vi "_012.vi"() -> ()   [LabVIEW 2024]
panel:
  out "output array":dbl[](array[numeric])
  in  "dimension size 2":i32
  in  "array 3":dbl[](array[numeric])
  out "min value":dbl
  out "max index(es)":i32
  out "min index(es)":i32
  out "max value":dbl
  in  "array 2":dbl[](array[numeric])
  out "subarray":dbl[](array[numeric])
  in  "length":i32
  in  "index":i32
  in  "array":dbl[](array[numeric])
  in  "element":dbl
  in  "element":dbl
  in  "element":dbl
  out "appended array":dbl[](array[numeric])
  in  "element":dbl
  out "initialized array":dbl[](array[numeric])
  in  "dimension size":i32
  in  "element":dbl
  # "Array :"
  # "Initilaize Array :"
  # "Build Array :"
  # "Array Subset :"
  # "Reshape Array :"
  # "Array Max & Min :"
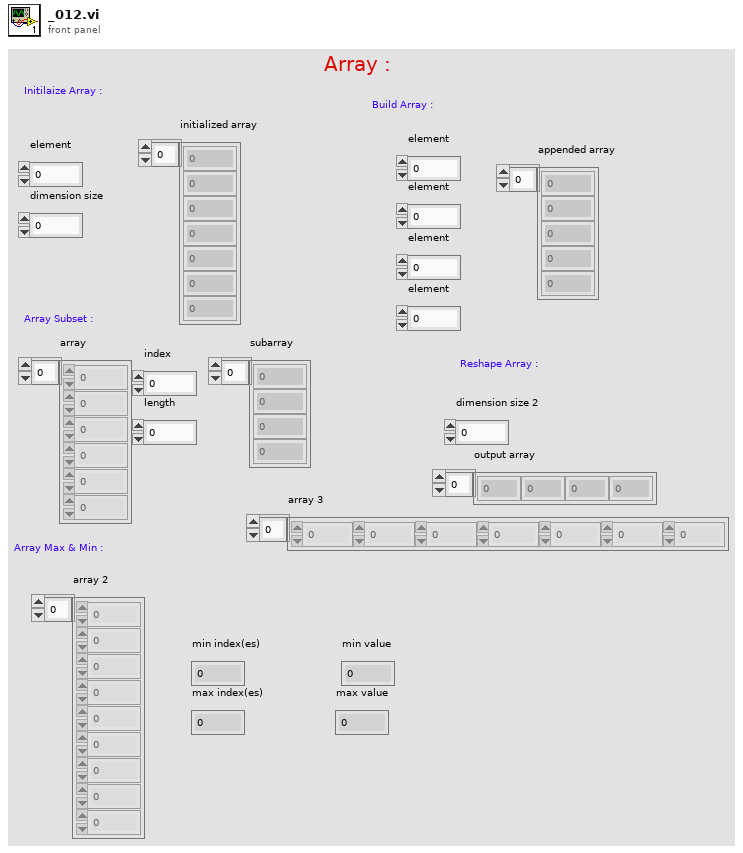
[diagram p1: front panel]
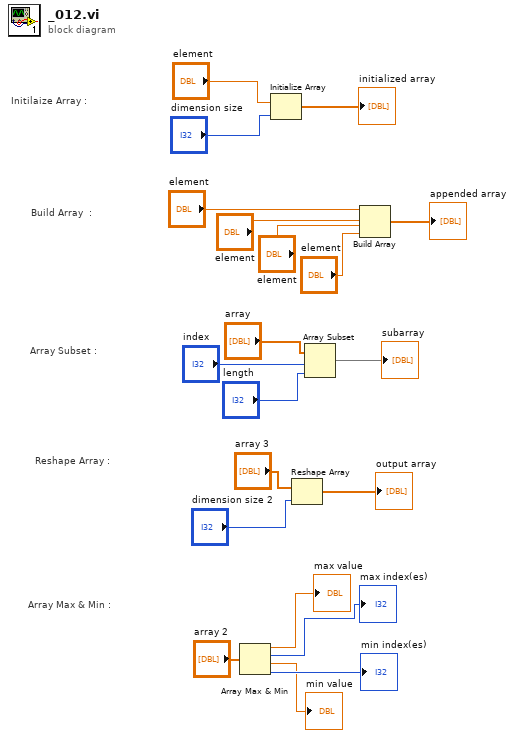
[diagram p0: block diagram]
diagram:
  # "Array Subset :"
  # "Array Max & Min :"
  # "Reshape Array :"
  # "Build Array  :"
  # "Initilaize Array :"
  n1 = Array Max & Min(array="array 2") -> (max value=→"max value":dbl, max index (indices)=→"max index(es)":i32, min value=→"min value":dbl, min index (indices)=→"min index(es)":i32)
  n2 = Initialize Array "Initialize Array"("element", "dimension size") -> (→"initialized array":dbl[])
  n3 = Reshape Array "Reshape Array"("array 3", "dimension size 2") -> (→"output array":dbl[])
  n4 = Array Subset "Array Subset"(array="array", index="index", length="length") -> (→"subarray":dbl[])
  n5 = Build Array "Build Array"("element", "element", "element", "element") -> (→"appended array":dbl[])
